vi "Baute Rate Calc.vi"(0 "Baud Rate (9600)":u32=9600, 9 "FPGA Clock Rate (40000000)":u32=40000000) -> (4 "Half Bit":u32, 6 "One Bit":u32, 8 "One and Half Bit":u32, 10 "Two Bit":u32)   [LabVIEW 2019, in "UART 8N1 (FPGA).lvlib"]
uses:
  UART 8N1 (FPGA).lvlib
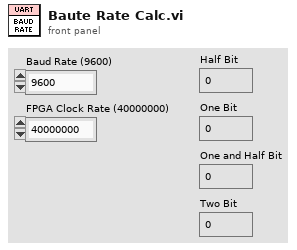
[diagram p1: front panel]
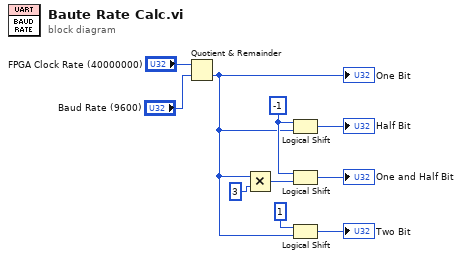
[diagram p0: block diagram]
diagram:
  w8 = i16 -1 ("y")
  n1 = Quotient & Remainder(x="FPGA Clock Rate (40000000)", y="Baud Rate (9600)") -> (floor(x/y)=w4:u32)  [unwired: 1 out]
  "One Bit" <- w4
  n2 = Multiply(x=w4, y=u32 3) -> (x*y=w10:u32)
  n3 = Logical Shift(y=w8, x=w4) -> (x << y=→"Half Bit":u32)
  n4 = Logical Shift(y=w8, x=w10) -> (x << y=→"One and Half Bit":u32)
  n5 = Logical Shift(y=i16 1, x=w4) -> (x << y=→"Two Bit":u32)
